vi "Begin.vi"(8 "error in (no error)":errorcluster, 11 "DriveMotorsRight in":refnum<class "DriveMotorsRight.lvclass">) -> (0 "error out":errorcluster, 3 "DriveMotorsRight out":refnum<class "DriveMotorsRight.lvclass">)   [LabVIEW 2013, in "DriveMotorsRight.lvclass"]
uses:
  DriveMotorsRight.lvclass
  DriveMotors/DriveMotors.lvclass
  <vilib>/Rock Robotics/WPI/MotorControl/WPI_MotorControlOpenCANJaguar.vi
panel:
  in  "Invert Motors":bool=TRUE
  in  "Motor3Can 2":u8=13
  in  "Motor2Can":u8=12
  in  "Motor1CAN":u8=11
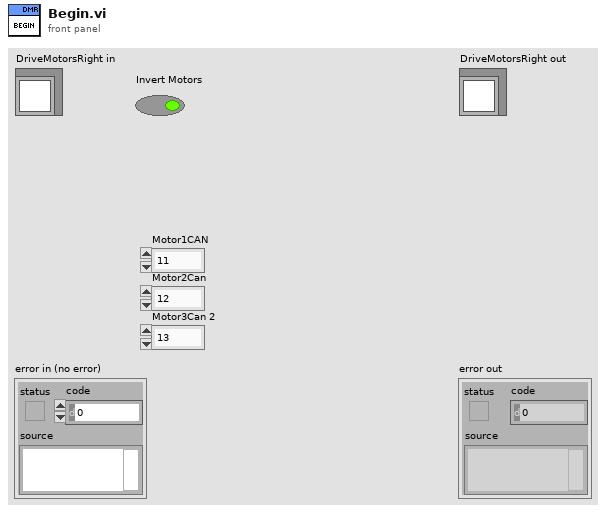
[diagram p1: front panel]
types:
  T1 = typedef "WPI_MotorControlDeviceRef.ctl" = cluster{"DeviceStatus":errorcluster, "Type":enum16{"PWM", "CAN"}, "PWM":cluster{"Digital Module":T2, "PWM Channel":T3, "DeadBand":T4}, "CAN":cluster{"Device Number":u8, "Control Mode":T5, "Semaphore":T6, "Max Vout":dbl}, "Invert":bool, "TransformRef":T7, "InvTransformRef":T7}
  T2 = typedef "FPGA_TypedefDigitalModule.ctl" = enum16{"Digital Module 1", "Digital Module 2"}
  T3 = typedef "FPGA_DIOPWMChannel.ctl" = enum8{"PWM 1", "PWM 2", "PWM 3", "PWM 4", "PWM 5", "PWM 6", "PWM 7", "PWM 8", "PWM 9", "PWM 10", "Invalid"}
  T4 = typedef "WPI_PWMDeadband.ctl" = cluster{"Name":string, "maxPositivePwm":i32, "minPositivePwm":i32, "centerPwm":i32, "maxNegativePwm":i32, "minNegativePwm":i32, "angularRange":u16}
  T5 = typedef "WPI_CANJaguar_ControlMode.ctl" = enum8{"Percent VBus", "Current", "Speed", "Position", "Voltage"}
  T6 = typedef "Semaphore RefNum" = refnum<k1>
  T7 = typedef "WPI_PWMTransform_ConPane.ctl" = refnum<vi>
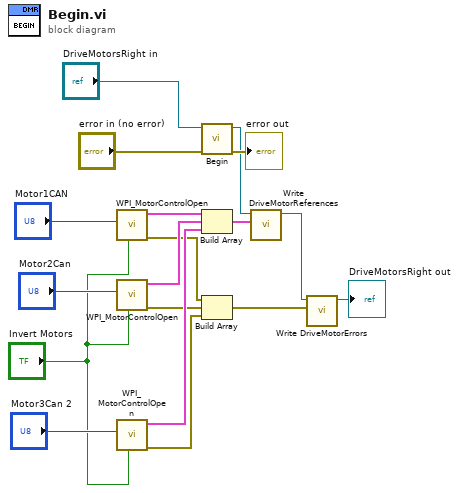
[diagram p0: block diagram]
diagram:
  n1 = call-poly <vilib>:"WPI_MotorControlOpen.vi"("Invert"="Invert Motors", "Device Number"="Motor1CAN") -> ("error out"=w3:errorcluster, "MotorControlDeviceRef"=w15:T1)  [unwired: 8 in]
  n2 = call-poly <vilib>:"WPI_MotorControlOpen.vi"("Invert"="Invert Motors", "Device Number"="Motor2Can") -> ("error out"=w2:errorcluster, "MotorControlDeviceRef"=w11:T1)  [unwired: 8 in]
  n3 = call-poly <vilib>:"WPI_MotorControlOpen.vi"("Invert"="Invert Motors", "Device Number"="Motor3Can 2") -> ("error out"=w1:errorcluster, "MotorControlDeviceRef"=w10:T1)  [unwired: 8 in]
  n4 = call-parent "Begin.vi"("error in (no error)"="error in (no error)", "DriveMotors in"="DriveMotorsRight in") -> ("error out"=→"error out":errorcluster, "DriveMotors out"=w9:refnum<class "DriveMotorsRight.lvclass">)  [unwired: 8 in]
  n5 = Build Array(w15, w11, w10) -> (w8:T1[])
  n6 = Build Array(w3, w2, w1) -> (w4:errorcluster[])
  n7 = call-dynamic "Write DriveMotorReferences.vi"("DriveMotorReferences"=w8, "DriveMotors in"=w9) -> ("DriveMotors out"=w6:refnum<class "DriveMotorsRight.lvclass">)  [unwired: 8 in, 1 out]
  n8 = call-dynamic "Write DriveMotorErrors.vi"("DriveMotorErrors"=w4, "DriveMotors in"=w6) -> ("DriveMotors out"=→"DriveMotorsRight out":refnum<class "DriveMotorsRight.lvclass">)  [unwired: 8 in, 1 out]
